vi "ExnSpectralBlock Spectral Measurements.vi"(0 "Signals":dynamicdata(graph), 1 "Selected Measurements":u32, 5 "Restart Averaging":bool, 7 "View":T2={"dB On (F)"=TRUE, "unwrap phase (F)"=FALSE, "convert to degree (F)"=FALSE}, 9 "Spectrum Window":u16=1, 11 "error in (no error)":errorcluster, 12 "Spectrum Averaging Parameters":T1={"averaging mode"=0, "weighting mode"=1, "number of averages"=10}, 14 "All Spectra":bool=TRUE) -> (4 "Measurement Output":dynamicdata(graph), 6 "averaging done":bool, 10 "Phase":dynamicdata(graph), 15 "error out":errorcluster)   [LabVIEW 2020]
doc: "Performs FFT-based spectral measurements, such as the averaged magnitude spectrum, power spectrum, and phase spectrum on a signal."
uses:
  <vilib>/measure/maspectr.llb/FFT Spectrum (Mag-Phase).vi
  <vilib>/measure/maspectr.llb/FFT Power Spectrum.vi
  <vilib>/measure/maspectr.llb/FFT Power Spectral Density.vi
  <vilib>/measure/NI_MAPro.lvlib
panel:
  in  "string":string=" Phase"
  in  "Array":string[](array[string])=["FFT - (RMS)", "FFT - (Peak)", "Power Spectrum", "PSD"]
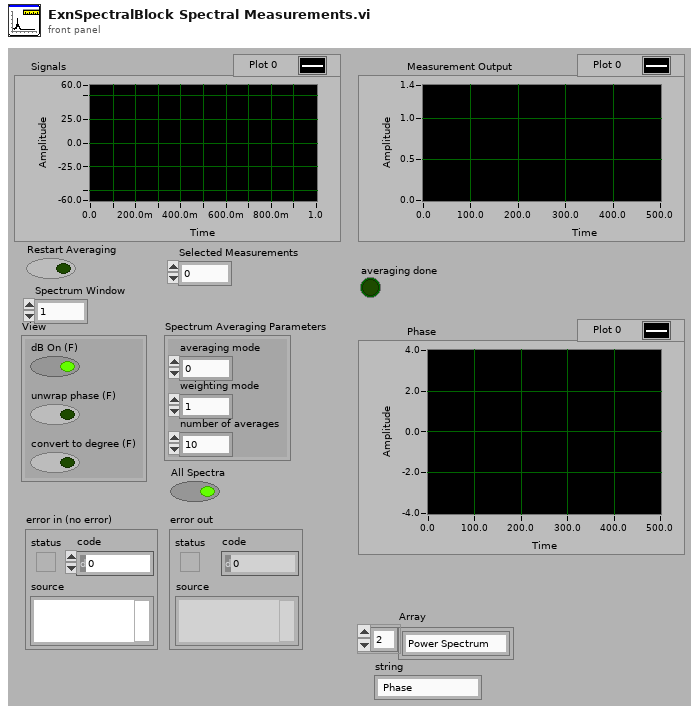
[diagram p1: front panel]
types:
  T1 = cluster{"averaging mode":u16, "weighting mode":u16, "number of averages":u32}
  T2 = cluster{"dB On (F)":bool, "unwrap phase (F)":bool, "convert to degree (F)":bool}
  T3 = enum16{"None ", "Hanning", "Hamming", "Blackman-Harris", "Exact Blackman", "Blackman", "Flat Top", "4 Term B-Harris ", "7 Term B-Harris", "Low Sidelobe"}
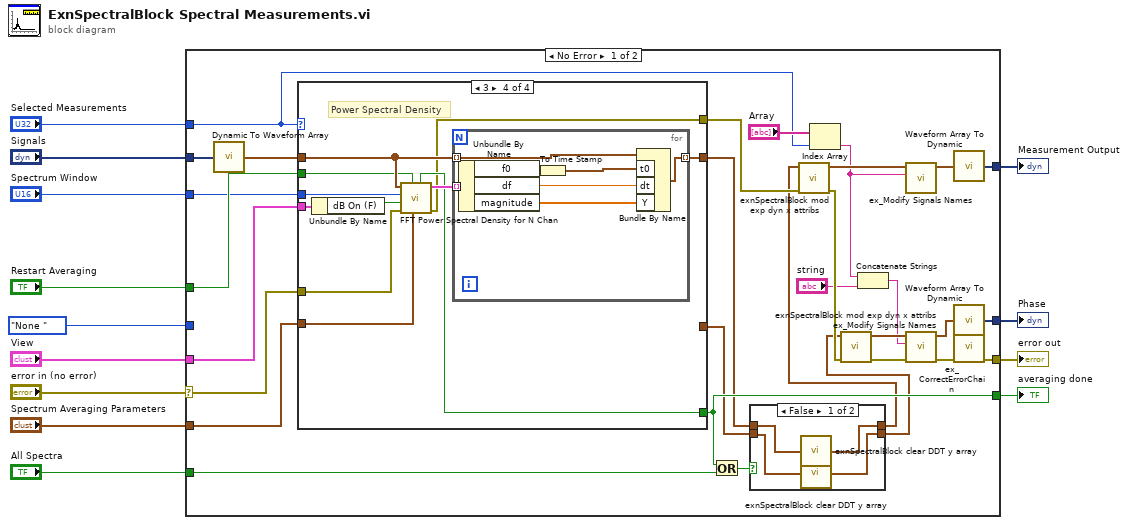
[diagram p0: block diagram]
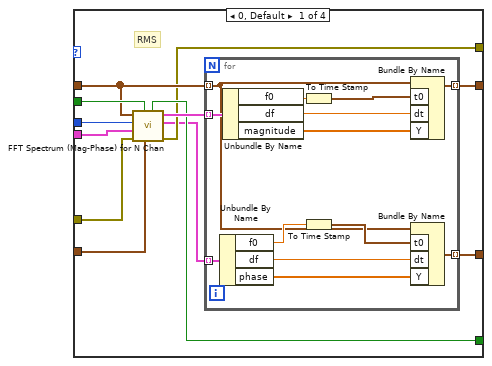
[diagram p3: hidden frame]
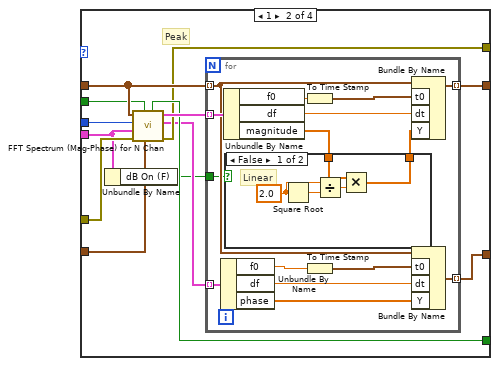
[diagram p4: hidden frame]
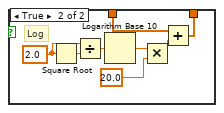
[diagram p5: hidden frame]
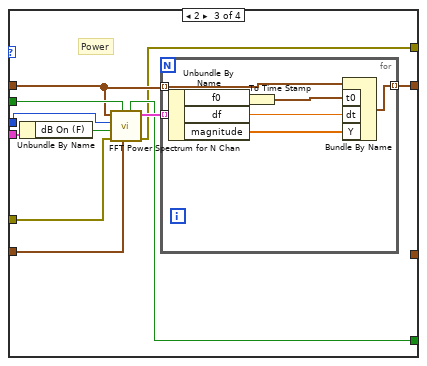
[diagram p6: hidden frame]
diagram:
  n1 = case shown="No Error" "error in (no error)" {
    selector: "error in (no error)" -> [w14 w152]
    tunnel: [w43 _] -> w13
    tunnel: [w42 _] -> w12
    tunnel: [w41 _] -> w11
    tunnel: "All Spectra" -> [w40 _]
    tunnel: "Spectrum Averaging Parameters" -> [w39 _]
    tunnel: "Restart Averaging" -> [w38 _]
    tunnel: T3."None " ("window") -> [_ _]
    tunnel: "Spectrum Window" -> [w15 _]
    tunnel: "View" -> [w36 _]
    tunnel: "Signals" -> [w34 _]
    tunnel: [w33 w152] -> w3
    tunnel: "Selected Measurements" -> [w25 _]
    frame No Error {
      n2 = call <vilib>:"Dynamic To Waveform Array.vi"("Input"=w34) -> ("Output"=w16:waveform(dbl)[])  [unwired: 4 out]
      n3 = case shown="3" w25 {
        tunnel: w16 -> [w56 w86 w123 w140]
        tunnel: [w61 w87 w126 w144] -> w19
        tunnel: w39 -> [w58 w84 w125 w139]
        tunnel: w36 -> [w59 w76 w121 w142]
        tunnel: w38 -> [w60 w85 w124 w138]
        tunnel: [w55 w82 w119 w137] -> w41
        tunnel: w15 -> [w54 w81 w118 w136]
        tunnel: w14 -> [w53 w79 w116 w135]
        tunnel: [w52 w80 w117 w134] -> w35
        tunnel: [w50 w78 _ _] -> w20
        frame 0, Default {
          # "RMS"
          n4 = call-poly <vilib>:"FFT Spectrum (Mag-Phase) for N Chan.vi"("averaging parameters"=w58, "restart averaging (F)"=w60, "error in (no error)"=w53, "view"=w59, "window"=w54, "time signals"=w56) -> ("error out"=w52:errorcluster, "phases"=w51:cluster{"f0":dbl, "df":dbl, "phase":dbl[]}[], "magnitudes"=w57:cluster{"f0":dbl, "df":dbl, "magnitude":dbl[]}[], "averaging done"=w55:bool)  [unwired: 1 in, 1 out]
          n5 = for {
            tunnel: w56 -> [w64] mode=indexing
            tunnel: [w71] -> w61 mode=indexing
            tunnel: w57 -> [w70] mode=indexing
            tunnel: w51 -> [w63] mode=indexing
            tunnel: [w62] -> w50 mode=indexing
            n6 = Unbundle By Name(w63) -> ("f0"=w67:dbl, "df"=w66:dbl, "phase"=w65:dbl[])
            n7 = Unbundle By Name(w70) -> ("f0"=w72:dbl, "df"=w73:dbl, "magnitude"=w74:dbl[])
            n8 = To Time Stamp(1:w72) -> (0:w69:timestamp)
            n9 = To Time Stamp(1:w67) -> (0:w68:timestamp)
            n10 = Bundle By Name(cluster=w64, "t0"=w69, "dt"=w73, "Y"=w74) -> (w71:waveform(dbl))
            n11 = Bundle By Name(cluster=w64, "t0"=w68, "dt"=w66, "Y"=w65) -> (w62:waveform(dbl))
          }
        }
        frame 1 {
          # "Peak"
          n12 = Unbundle By Name(w76) -> ("dB On (F)"=w75:bool)
          n13 = call-poly <vilib>:"FFT Spectrum (Mag-Phase) for N Chan.vi"("averaging parameters"=w84, "restart averaging (F)"=w85, "error in (no error)"=w79, "view"=w76, "window"=w81, "time signals"=w86) -> ("error out"=w80:errorcluster, "phases"=w77:cluster{"f0":dbl, "df":dbl, "phase":dbl[]}[], "magnitudes"=w83:cluster{"f0":dbl, "df":dbl, "magnitude":dbl[]}[], "averaging done"=w82:bool)  [unwired: 1 in, 1 out]
          n14 = for {
            tunnel: w86 -> [w91] mode=indexing
            tunnel: [w100] -> w87 mode=indexing
            tunnel: w83 -> [w99] mode=indexing
            tunnel: [w90] -> w78 mode=indexing
            tunnel: w77 -> [w89] mode=indexing
            tunnel: w75 -> [w88]
            n15 = Unbundle By Name(w89) -> ("f0"=w94:dbl, "df"=w93:dbl, "phase"=w92:dbl[])
            n16 = Unbundle By Name(w99) -> ("f0"=w101:dbl, "df"=w102:dbl, "magnitude"=w98:dbl[])
            n17 = case shown="False" w88 {
              tunnel: w98 -> [w106 w115]
              tunnel: [w105 w114] -> w97
              frame False {
                w104 = 2.0 ("y")
                # "Linear"
                n18 = Square Root(x=w104) -> (sqrt(x)=w107:dbl)
                n19 = Divide(x=w104, y=w107) -> (x/y=w103:dbl)
                n20 = Multiply(x=w106, y=w103) -> (x*y=w105:dbl[])
              }
              frame True {
                w112 = 2.0 ("y")
                # "Log"
                n21 = Square Root(x=w112) -> (sqrt(x)=w113:dbl)
                n22 = Divide(x=w112, y=w113) -> (x/y=w110:dbl)
                n23 = Logarithm Base 10(1:w110) -> (0:w108:dbl)
                n24 = Multiply(x=w108, y=20.0) -> (x*y=w109:dbl)
                n25 = Add(x=w115, y=w109) -> (x+y=w114:dbl[])
              }
            }
            n26 = To Time Stamp(1:w101) -> (0:w96:timestamp)
            n27 = To Time Stamp(1:w94) -> (0:w95:timestamp)
            n28 = Bundle By Name(cluster=w91, "t0"=w96, "dt"=w102, "Y"=w97) -> (w100:waveform(dbl))
            n29 = Bundle By Name(cluster=w91, "t0"=w95, "dt"=w93, "Y"=w92) -> (w90:waveform(dbl))
          }
        }
        frame 2 {
          # "Power"
          n30 = Unbundle By Name(w121) -> ("dB On (F)"=w120:bool)
          n31 = call-poly <vilib>:"FFT Power Spectrum for N Chan.vi"("averaging parameters"=w125, "restart averaging (F)"=w124, "error in (no error)"=w116, "dB On (F)"=w120, "window"=w118, "time signals"=w123) -> ("error out"=w117:errorcluster, "power spectra"=w122:cluster{"f0":dbl, "df":dbl, "magnitude":dbl[]}[], "averaging done"=w119:bool)  [unwired: 3 out]
          n32 = for {
            tunnel: w123 -> [w131] mode=indexing
            tunnel: [w130] -> w126 mode=indexing
            tunnel: w122 -> [w128] mode=indexing
            n33 = Unbundle By Name(w128) -> ("f0"=w132:dbl, "df"=w133:dbl, "magnitude"=w129:dbl[])
            n34 = To Time Stamp(1:w132) -> (0:w127:timestamp)
            n35 = Bundle By Name(cluster=w131, "t0"=w127, "dt"=w133, "Y"=w129) -> (w130:waveform(dbl))
          }
        }
        frame 3 {
          # "Power Spectral Density"
          n36 = Unbundle By Name(w142) -> ("dB On (F)"=w143:bool)
          n37 = call-poly <vilib>:"FFT Power Spectral Density for N Chan.vi"("averaging parameters"=w139, "restart averaging (F)"=w138, "error in (no error)"=w135, "dB On (F)"=w143, "window"=w136, "time signals"=w140) -> ("error out"=w134:errorcluster, "power spectral densities"=w141:cluster{"f0":dbl, "df":dbl, "magnitude":dbl[]}[], "averaging done"=w137:bool)  [unwired: 3 out]
          n38 = for {
            tunnel: w140 -> [w147] mode=indexing
            tunnel: [w148] -> w144 mode=indexing
            tunnel: w141 -> [w146] mode=indexing
            n39 = Unbundle By Name(w146) -> ("f0"=w151:dbl, "df"=w150:dbl, "magnitude"=w149:dbl[])
            n40 = To Time Stamp(1:w151) -> (0:w145:timestamp)
            n41 = Bundle By Name(cluster=w147, "t0"=w145, "dt"=w150, "Y"=w149) -> (w148:waveform(dbl))
          }
        }
      }
      n42 = Or(x=w41, y=w40) -> (x .or. y?=w21:bool)
      n43 = case shown="False" w21 {
        tunnel: w20 -> [w45 w48]
        tunnel: w19 -> [w47 w49]
        tunnel: [w46 w49] -> w18
        tunnel: [w44 w48] -> w17
        frame False {
          n44 = call <vilib>:"exnSpectralBlock clear DDT y array.vi"("Array In"=w47) -> ("Array Out"=w46:waveform(dbl)[])
          n45 = call <vilib>:"exnSpectralBlock clear DDT y array.vi"("Array In"=w45) -> ("Array Out"=w44:waveform(dbl)[])
        }
        frame True {
        }
      }
      n46 = call <vilib>:"exnSpectralBlock mod exp dyn x attribs.vi"("error in (no error)"=w35, "Signals in"=w18) -> ("error out"=w37:errorcluster, "Signals out"=w32:waveform(dbl)[])  [unwired: 2 in, 6 out]
      n47 = Index Array(array="Array", index=w25) -> (element=w24:string)
      n48 = call <vilib>:"exnSpectralBlock mod exp dyn x attribs.vi"("error in (no error)"=w37, "Signals in"=w17) -> ("error out"=w30:errorcluster, "Signals out"=w27:waveform(dbl)[])  [unwired: 2 in, 6 out]
      n49 = Concatenate Strings(w24, "string") -> (w22:string)
      n50 = call <vilib>:"ex_Modify Signals Names.vi"("Name Modifier"=w24, "Array of Waveforms In"=w32) -> ("Array of Waveforms Out"=w31:waveform(dbl)[])  [unwired: 1 in, 8 out]
      n51 = call <vilib>:"ex_Modify Signals Names.vi"("error in (no error)"=w30, "Name Modifier"=w22, "Array of Waveforms In"=w27) -> ("error out"=w29:errorcluster, "Array of Waveforms Out"=w28:waveform(dbl)[])  [unwired: 7 out]
      n52 = call <vilib>:"Waveform Array To Dynamic.vi"("Input"=w31) -> ("Output"=w43:dynamicdata)  [unwired: 4 out]
      n53 = call <vilib>:"Waveform Array To Dynamic.vi"("Input"=w28) -> ("Output"=w42:dynamicdata)  [unwired: 4 out]
      n54 = call <vilib>:"ex_CorrectErrorChain.vi"("error in (no error)"=w29) -> ("error out"=w33:errorcluster)  [unwired: 1 in, 9 out]
    }
    frame Error {
    }
  }
  "Phase" <- w12
  "Measurement Output" <- w13
  "averaging done" <- w11
  "error out" <- w3
